vi "CheckChecksum.vi"(11 "String":string) -> (2 "Checksum Received":string, 3 "x = y?":bool)   [LabVIEW 2015]
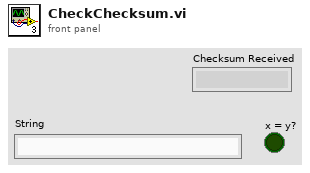
[diagram p1: front panel]
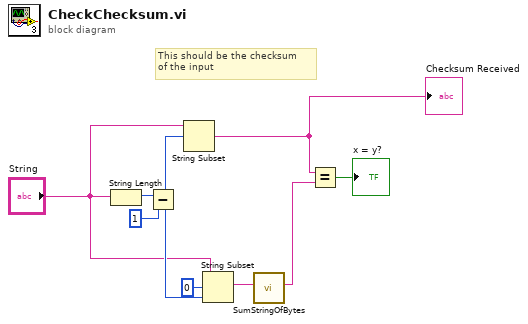
[diagram p0: block diagram]
diagram:
  # "This should be the checksum \nof the input"
  n1 = String Length(string="String") -> (length=w9:i32)
  n2 = Subtract(x=w9, y=1) -> (x-y=w3:i32)
  n3 = String Subset(string="String", offset (0)=w3) -> (substring=w6:string)  [unwired: 1 in]
  "Checksum Received" <- w6
  n4 = String Subset(string="String", offset (0)=0, length (rest)=w3) -> (substring=w7:string)
  n5 = call "SumStringOfBytes.vi"("String Of Bytes"=w7) -> ("SumAsString"=w5:string)  [unwired: 10 in]
  n6 = Equal?(x=w6, y=w5) -> (x = y?=→"x = y?":bool)
